vi "Login to Station.vi"(8 "error in (no error)":errorcluster) -> (0 "error out":errorcluster, 2 "Logged In":bool)   [LabVIEW 2016]
uses:
  <vilib>/Instr/_visa.llb/VISA Configure Serial Port (Instr).vi
  controls/Save Path Control.ctl
  Message Queue/Message Cluster.ctl
  Message Queue/GLDL Message Queue.lvlib
  Message Queue/All Message Queues.ctl
  controls/Connected Indicator.ctl
  controls/Output Indicator.ctl
  controls/Disconnect Control.ctl
  controls/Download Control.ctl
  controls/Exit Control.ctl
  controls/Date Control.ctl
  controls/COM Port Control.ctl
  controls/IP Phone Number Control.ctl
  controls/GLDL UI Data.ctl
panel:
  out "Data Cluster In 2":T1
  in  "Data Cluster In":T1
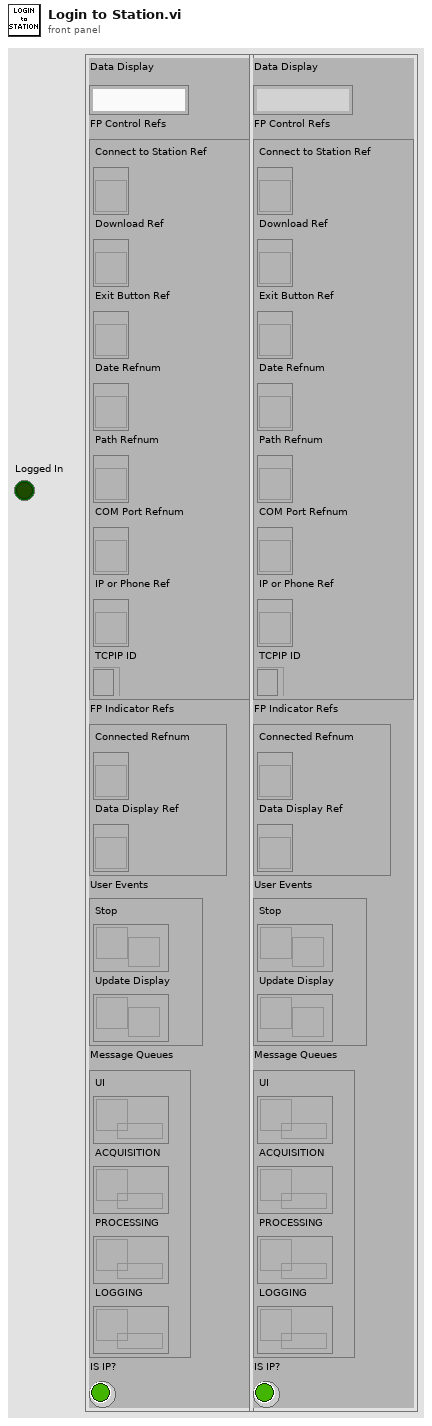
[diagram p1: front panel]
types:
  T1 = typedef "GLDL UI Data.ctl" = cluster{"Data Display":string, "FP Control Refs":cluster{"Connect to Station Ref":refnum<vi>, "Download Ref":refnum<vi>, "Exit Button Ref":refnum<vi>, "Date Refnum":refnum<vi>, "Path Refnum":refnum<vi>, "COM Port Refnum":refnum<vi>, "IP or Phone Ref":refnum<vi>, "TCPIP ID":refnum<k5>}, "FP Indicator Refs":cluster{"Connected Refnum":refnum<vi>, "Data Display Ref":refnum<vi>}, "User Events":cluster{"Stop":refnum<user-event>, "Update Display":refnum<user-event>}, "Message Queues":T2, "IS IP?":bool}
  T2 = typedef "GLDL Message Queue.lvlib/All Message Queues.ctl" = cluster{"UI":refnum<queue>, "ACQUISITION":refnum<queue>, "PROCESSING":refnum<queue>, "LOGGING":refnum<queue>}
  T3 = enum16{"Standard", "Buffered", "CRLF", "Immediate"}
  T4 = typedef "Output Indicator.ctl" = string
  T5 = typedef "COM Port Control.ctl" = refnum<visa-resource-name>
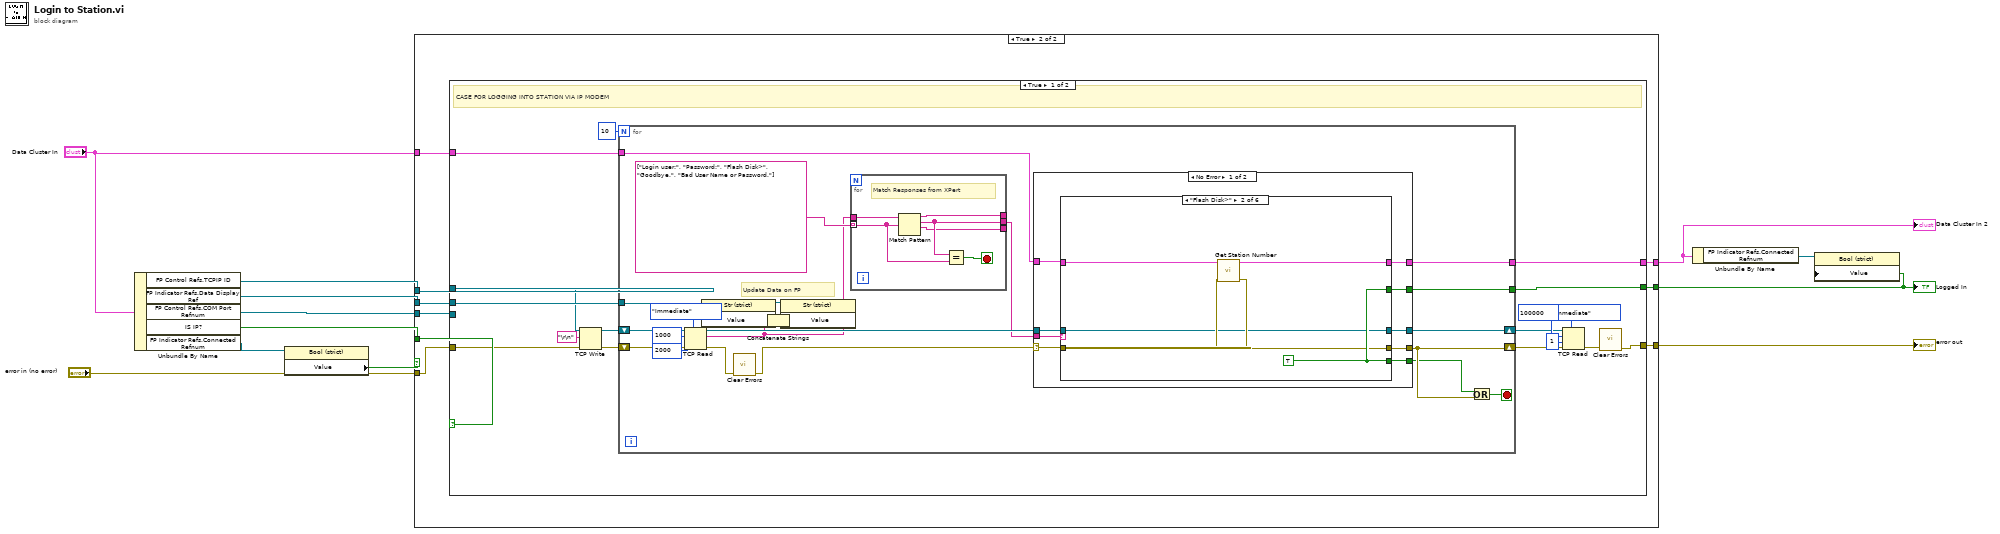
[diagram p0: block diagram]
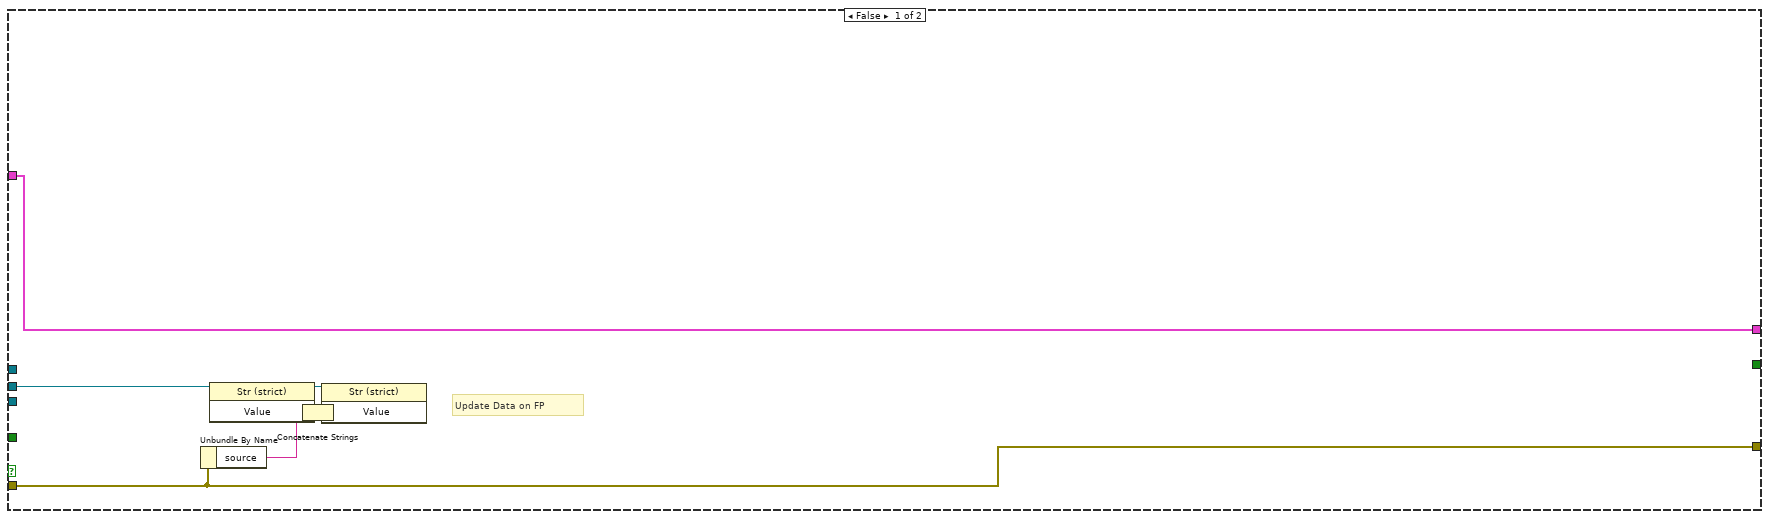
[diagram p2: hidden frame]
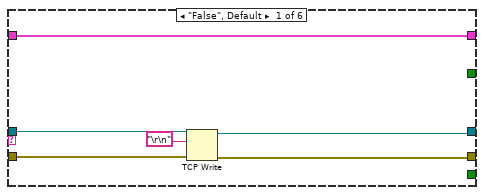
[diagram p3: hidden frame]
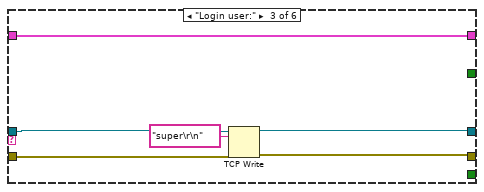
[diagram p4: hidden frame]
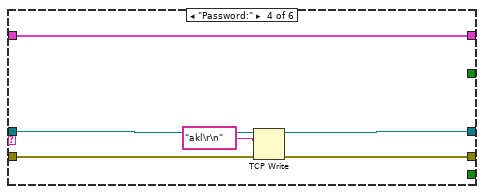
[diagram p5: hidden frame]
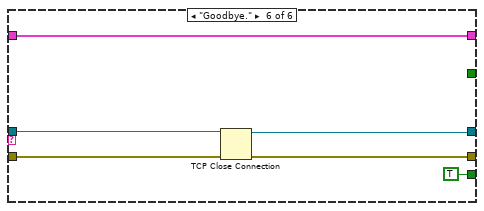
[diagram p7: hidden frame]
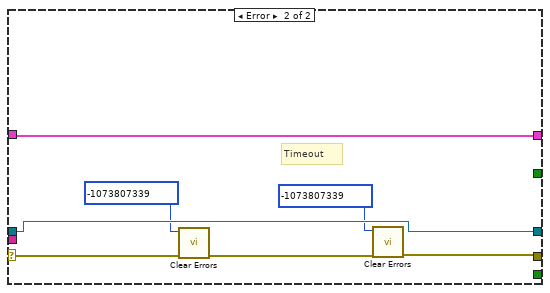
[diagram p8: hidden frame]
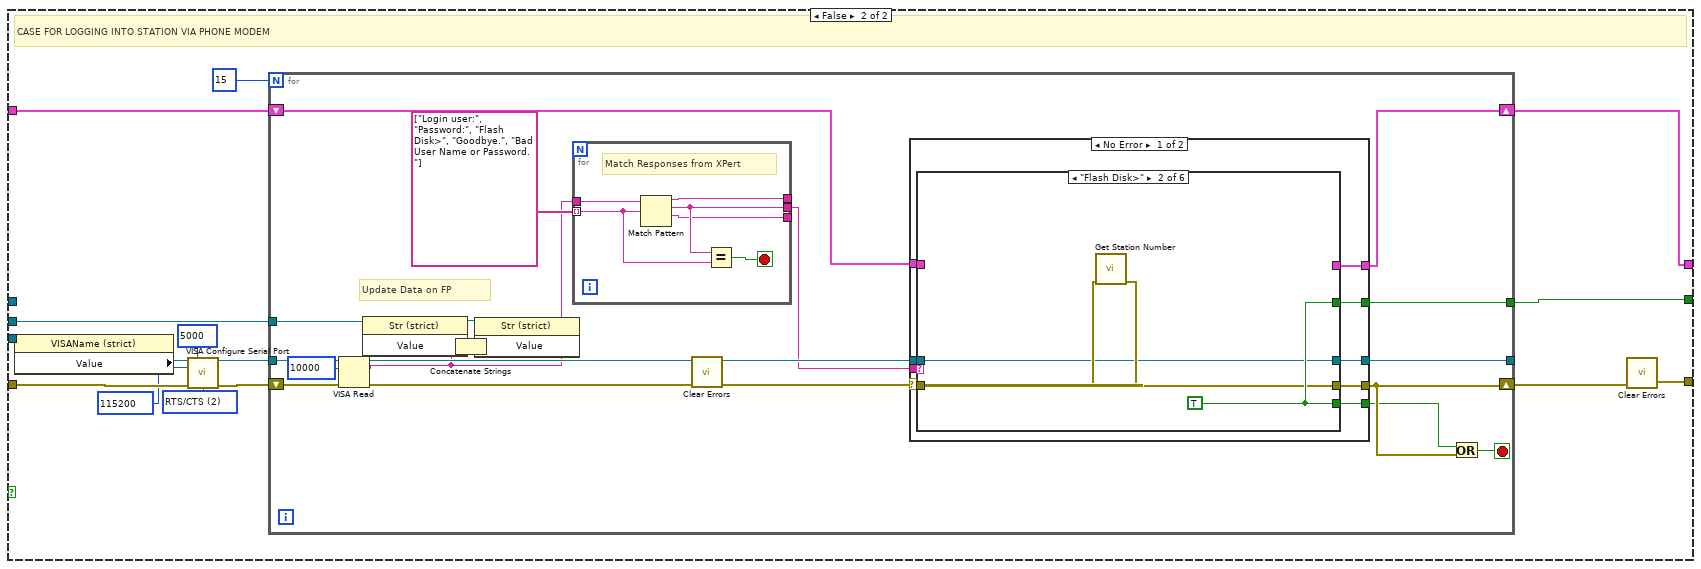
[diagram p9: hidden frame]
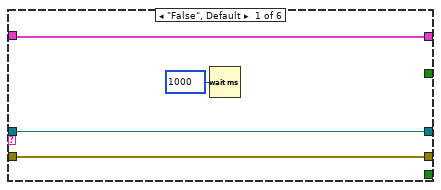
[diagram p10: hidden frame]
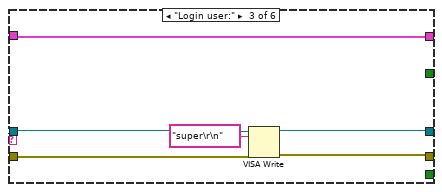
[diagram p11: hidden frame]
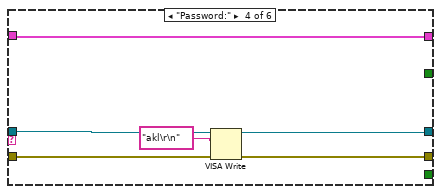
[diagram p12: hidden frame]
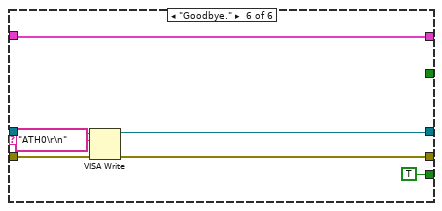
[diagram p14: hidden frame]
diagram:
  n1 = Unbundle By Name("Data Cluster In") -> ("FP Control Refs.TCPIP ID"=w10:refnum<k5>, "FP Indicator Refs.Data Display Ref"=w9:refnum<vi>, "FP Control Refs.COM Port Refnum"=w8:refnum<vi>, "IS IP?"=w7:bool, "FP Indicator Refs.Connected Refnum"=w6:refnum<vi>)
  n2 = property class="Bool (strict)"(reference=w6) -> ("Value"=w5:bool)  [unwired: 1 in, 2 out]
  n3 = case shown="True" w5 {
    tunnel: [w14 w28] -> w12
    tunnel: "error in (no error)" -> [w14 w27]
    tunnel: [_ w26] -> w3
    tunnel: w10 -> [_ w25]
    tunnel: w9 -> [w15 w24]
    tunnel: w8 -> [_ w23]
    tunnel: w7 -> [_ w22]
    tunnel: "Data Cluster In" -> [w19 w21]
    tunnel: [w19 w20] -> w1
    frame False {
      # "Update Data on FP"
      n4 = Unbundle By Name(w14) -> ("source"=w13:string)
      n5 = property class="Str (strict)"(reference=w15) -> (reference out=w18:refnum<vi>, "Value"=w16:T4)  [unwired: 1 in, 1 out]
      n6 = Concatenate Strings(w16, w13) -> (w17:string)
      n7 = property class="Str (strict)"(reference=w18, "Value"=w17) -> ()  [unwired: 1 in, 2 out]
    }
    frame True {
      n8 = case shown="True" w22 {
        tunnel: [w31 w134] -> w28
        tunnel: w27 -> [w38 w128]
        tunnel: w23 -> [_ w130]
        tunnel: [w44 w136] -> w26
        tunnel: w25 -> [w40 _]
        tunnel: w24 -> [w43 w135]
        tunnel: w21 -> [w30 w133]
        tunnel: [w29 w132] -> w20
        frame True {
          # "CASE FOR LOGGING INTO STATION VIA IP MODEM"
          n9 = TCP Write(connection ID=w40, data in="\r\n", error in (no error)=w38) -> (connection ID out=w41:refnum<k5>, error out=w39:errorcluster)  [unwired: 1 in, 1 out]
          n10 = for {
            N: 10 -> [_]
            shift-right: [w66] -> w32
            shift-left: w39 -> [w59]
            shift-right: [w67] -> w33
            shift-left: w41 -> [w58]
            tunnel: [w63] -> w44
            tunnel: w43 -> [w52]
            tunnel: w30 -> [w47]
            tunnel: [w46] -> w29
            stop <- w64 stop-if-true
            # "Update Data on FP"
            n11 = TCP Read(connection ID=w58, bytes to read=1000, error in (no error)=w59, 7:T3."Immediate" ("mode (standard)"), 9:2000 ("timeout ms (25000)")) -> (connection ID out=w61:refnum<k5>, data out=w50:string, error out=w54:errorcluster)
            n12 = property class="Str (strict)"(reference=w52) -> (reference out=w51:refnum<vi>, "Value"=w48:T4)  [unwired: 1 in, 1 out]
            n13 = call <vilib>:"Clear Errors.vi"("error in (no error)"=w54) -> ("error out"=w53:errorcluster)  [unwired: 5 in, 1 out]
            n14 = Concatenate Strings(w48, w50) -> (w49:string)
            n15 = property class="Str (strict)"(reference=w51, "Value"=w49) -> ()  [unwired: 1 in, 2 out]
            n16 = for {
              tunnel: string[] ["Login user:", "Password:", "Flash Disk>", "Goodbye.", "Bad User Name or Password."] -> [w70] mode=indexing
              tunnel: [w72] -> w56
              tunnel: w50 -> [w71]
              tunnel: [w69] -> _
              tunnel: [w68] -> _
              stop <- w73 stop-if-true
              # "Match Responses from XPert"
              n17 = Match Pattern(string=w71, regular expression=w70) -> (before substring=w68:string, match substring=w72:string, after substring=w69:string)  [unwired: 1 in, 1 out]
              n18 = Equal?(x=w72, y=w70) -> (x = y?=w73:bool)
            }
            n19 = case shown="No Error" w53 {
              selector: w53 -> [w79 w117]
              tunnel: w56 -> [w77 _]
              tunnel: w61 -> [w82 w121]
              tunnel: [w81 w121] -> w67
              tunnel: [w80 w122] -> w66
              tunnel: [w78 _] -> w65
              tunnel: [w76 _] -> w63
              tunnel: w47 -> [w75 w116]
              tunnel: [w74 w116] -> w46
              frame No Error {
                n20 = case shown="\"Flash Disk>\"" w77 {
                  tunnel: w79 -> [w85 w93 w98 w103 w108 w114]
                  tunnel: w82 -> [w88 w91 w99 w106 w109 w115]
                  tunnel: [w87 w91 w97 w105 w109 w113] -> w81
                  tunnel: [w86 w92 w96 w104 w108 w112] -> w80
                  tunnel: [_ w94 _ _ _ TRUE] -> w78
                  tunnel: [_ w94 _ _ _ _] -> w76
                  tunnel: w75 -> [w83 w89 w95 w101 w107 w110]
                  tunnel: [w83 w90 w95 w101 w107 w110] -> w74
                  frame "False", Default {
                    n21 = TCP Write(connection ID=w88, data in="\r\n", error in (no error)=w85) -> (connection ID out=w87:refnum<k5>, error out=w86:errorcluster)  [unwired: 1 in, 1 out]
                  }
                  frame "Flash Disk>" {
                    w94 = TRUE
                    n22 = call "Get Station Number.vi"("error in (no error)"=w93, "UI Data in"=w89) -> ("error out (no error)"=w92:errorcluster, "UI Data out"=w90:T1)  [unwired: 8 in]
                  }
                  frame "Login user:" {
                    n23 = TCP Write(connection ID=w99, data in="super\r\n" ("write buffer"), error in (no error)=w98) -> (connection ID out=w97:refnum<k5>, error out=w96:errorcluster)  [unwired: 1 in, 1 out]
                  }
                  frame "Password:" {
                    n24 = TCP Write(connection ID=w106, data in="akl\r\n" ("write buffer"), error in (no error)=w103) -> (connection ID out=w105:refnum<k5>, error out=w104:errorcluster)  [unwired: 1 in, 1 out]
                  }
                  frame "Bad User Name or Password." {
                  }
                  frame "Goodbye." {
                    n25 = TCP Close Connection(connection ID=w115, error in (no error)=w114) -> (connection ID out=w113:refnum<k5>, error out=w112:errorcluster)  [unwired: 1 in]
                  }
                }
              }
              frame Error {
                # "Timeout"
                n26 = call <vilib>:"Clear Errors.vi"("error in (no error)"=w117, "specific error code to clear (0: all)"=-1073807339) -> ("error out"=w118:errorcluster)  [unwired: 4 in, 1 out]
                n27 = call <vilib>:"Clear Errors.vi"("error in (no error)"=w118, "specific error code to clear (0: all)"=-1073807339) -> ("error out"=w122:errorcluster)  [unwired: 4 in, 1 out]
              }
            }
            n28 = Or(x=w65, y=w66) -> (x .or. y?=w64:bool)
          }
          n29 = TCP Read(connection ID=w33, bytes to read=100000, error in (no error)=w32, 7:T3."Immediate" ("mode (standard)"), 9:1 ("timeout ms (25000)")) -> (error out=w34:errorcluster)  [unwired: 2 out]
          n30 = call <vilib>:"Clear Errors.vi"("error in (no error)"=w34) -> ("error out"=w31:errorcluster)  [unwired: 5 in, 1 out]
        }
        frame False {
          w125 = u16 2 items=["None", "XON/XOFF", "RTS/CTS", "XON/XOFF & RTS/CTS", "DTR/DSR", "XON/XOFF & DTR/DSR"] ("flow control (0:none)")
          # "CASE FOR LOGGING INTO STATION VIA PHONE MODEM"
          n31 = property class="VISAName (strict)"(reference=w130) -> ("Value"=w129:T5)  [unwired: 1 in, 2 out]
          n32 = call-poly "VISA Configure Serial Port"("VISA resource name"=w129, "timeout (10sec)"=u32 5000, "baud rate (9600)"=u32 115200, "error in (no error)"=w128, "flow control (0:none)"=w125) -> ("VISA resource name out"=w126:refnum<visa-resource-name>, "error out"=w127:errorcluster)  [unwired: 9 in]
          n33 = for {
            N: 15 -> [_]
            shift-right: [w157] -> w131
            shift-left: w127 -> [w152]
            tunnel: [w154] -> w136
            tunnel: w135 -> [w147]
            shift-right: [w143] -> w132
            shift-left: w133 -> [w138]
            tunnel: w126 -> [w140]
            tunnel: [w139] -> _
            stop <- w155 stop-if-true
            # "Update Data on FP"
            n34 = VISA Read(VISA resource name=w140, byte count=u32 10000, error in (no error)=w152) -> (VISA resource name out=w153:refnum<visa-resource-name>, read buffer=w142:string, error out=w149:errorcluster)  [unwired: 1 out]
            n35 = property class="Str (strict)"(reference=w147) -> (reference out=w146:refnum<vi>, "Value"=w144:T4)  [unwired: 1 in, 1 out]
            n36 = Concatenate Strings(w144, w142) -> (w145:string)
            n37 = property class="Str (strict)"(reference=w146, "Value"=w145) -> ()  [unwired: 1 in, 2 out]
            n38 = for {
              tunnel: string[] ["Login user:", "Password:", "Flash Disk>", "Goodbye.", "Bad User Name or Password."] -> [w160] mode=indexing
              tunnel: [w162] -> w150
              tunnel: w142 -> [w161]
              tunnel: [w159] -> _
              tunnel: [w158] -> _
              stop <- w163 stop-if-true
              # "Match Responses from XPert"
              n39 = Match Pattern(string=w161, regular expression=w160) -> (before substring=w158:string, match substring=w162:string, after substring=w159:string)  [unwired: 1 in, 1 out]
              n40 = Equal?(x=w162, y=w160) -> (x = y?=w163:bool)
            }
            n41 = call <vilib>:"Clear Errors.vi"("error in (no error)"=w149) -> ("error out"=w148:errorcluster)  [unwired: 5 in, 1 out]
            n42 = case shown="No Error" w148 {
              selector: w148 -> [w170 w205]
              tunnel: w150 -> [w168 _]
              tunnel: w153 -> [w172 w203]
              tunnel: [w164 w203] -> w139
              tunnel: [w171 w205] -> w157
              tunnel: [w169 _] -> w156
              tunnel: [w167 _] -> w154
              tunnel: w138 -> [w166 w204]
              tunnel: [w165 w204] -> w143
              frame No Error {
                n43 = case shown="\"Flash Disk>\"" w168 {
                  tunnel: w170 -> [w175 w179 w184 w190 w195 w202]
                  tunnel: w172 -> [w176 w177 w185 w192 w193 w196]
                  tunnel: [w175 w178 w183 w191 w195 w201] -> w171
                  tunnel: [_ w180 _ _ _ TRUE] -> w169
                  tunnel: [_ w180 _ _ _ _] -> w167
                  tunnel: w166 -> [w174 _ w182 w188 w194 w199]
                  tunnel: [w174 _ w182 w188 w194 w199] -> w165
                  tunnel: [w176 w177 w181 w187 w193 w198] -> w164
                  frame "False", Default {
                    n44 = Wait (ms)(milliseconds to wait=u32 1000) -> ()  [unwired: 1 out]
                  }
                  frame "Flash Disk>" {
                    w180 = TRUE
                    n45 = call "Get Station Number.vi"("error in (no error)"=w179) -> ("error out (no error)"=w178:errorcluster)  [unwired: 9 in, 1 out]
                  }
                  frame "Login user:" {
                    n46 = VISA Write(VISA resource name=w185, write buffer="super\r\n", error in (no error)=w184) -> (VISA resource name out=w181:refnum<visa-resource-name>, error out=w183:errorcluster)  [unwired: 1 out]
                  }
                  frame "Password:" {
                    n47 = VISA Write(VISA resource name=w192, write buffer="akl\r\n", error in (no error)=w190) -> (VISA resource name out=w187:refnum<visa-resource-name>, error out=w191:errorcluster)  [unwired: 1 out]
                  }
                  frame "Bad User Name or Password." {
                  }
                  frame "Goodbye." {
                    n48 = VISA Write(VISA resource name=w196, write buffer="ATH0\r\n", error in (no error)=w202) -> (VISA resource name out=w198:refnum<visa-resource-name>, error out=w201:errorcluster)  [unwired: 1 out]
                  }
                }
              }
              frame Error {
              }
            }
            n49 = Or(x=w156, y=w157) -> (x .or. y?=w155:bool)
          }
          n50 = call <vilib>:"Clear Errors.vi"("error in (no error)"=w131) -> ("error out"=w134:errorcluster)  [unwired: 5 in, 1 out]
        }
      }
    }
  }
  "error out" <- w12
  "Logged In" <- w3
  "Data Cluster In 2" <- w1
  n51 = Unbundle By Name(w1) -> ("FP Indicator Refs.Connected Refnum"=w4:refnum<vi>)
  n52 = property class="Bool (strict)"(reference=w4, "Value"=w3) -> ()  [unwired: 1 in, 2 out]
